vi "Redo.vi"(8 "error in (no error)":errorcluster, 11 "UndoObject in":refnum<class "UndoObject.lvclass">) -> (0 "error out":errorcluster, 2 "Ctrl Val.Get All":T1[](array[typedef]), 3 "UndoObject out":refnum<class "UndoObject.lvclass">, 4 "Redo Enable":bool, 6 "Undo Enable":bool)   [LabVIEW 2015, in "UndoLibrary.lvlib" / "UndoObject.lvclass"]
doc: "This VI stores the values to perform the redo action."
uses:
  UndoObject.lvclass
  Support VIs/DataClass/Controls/cluster_Control Value.ctl
  UndoObject.lvclass/UndoObject.ctl
  Support VIs/DataClass/DataObject.lvclass/DataObject.ctl
  QueueOperations/QueueOperations.lvlib
  Support VIs/DataClass/DataObject.lvclass
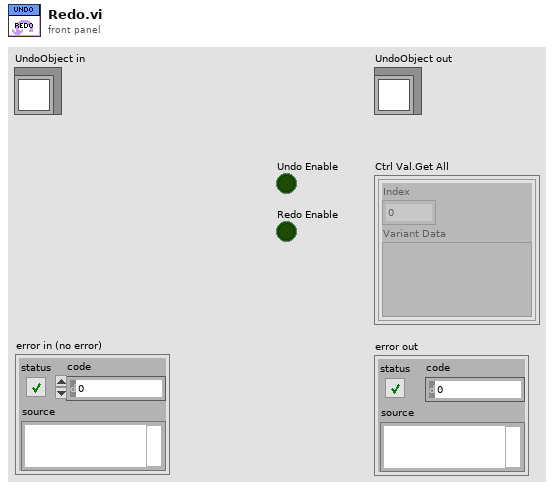
[diagram p1: front panel]
types:
  T1 = typedef "UndoLibrary.lvlib/DataObject.lvclass/cluster_Control Value.ctl" = cluster{"Index":i32, "Variant Data":variant}
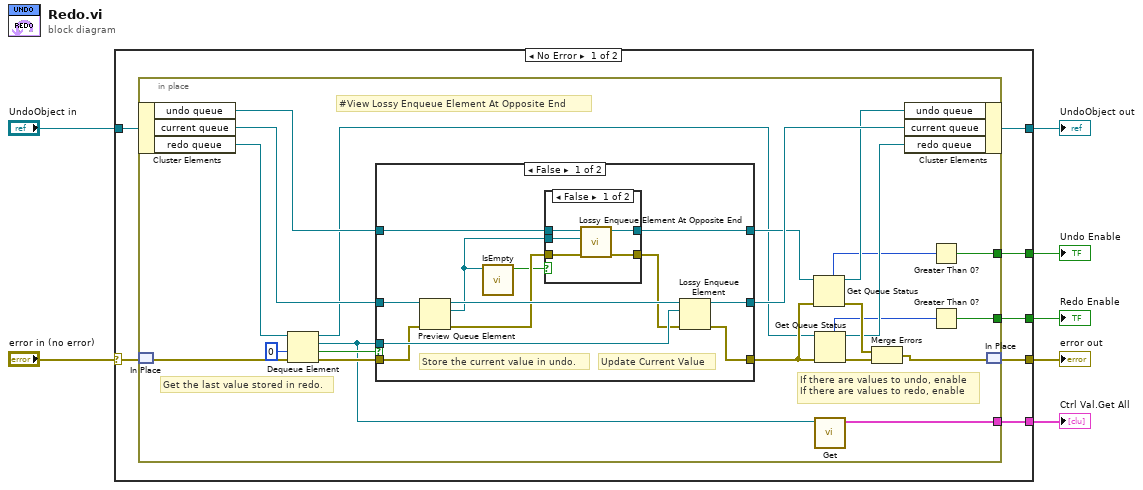
[diagram p0: block diagram]
diagram:
  n1 = case shown="No Error" "error in (no error)" {
    selector: "error in (no error)" -> [w13 w60]
    tunnel: [w12 w60] -> w7
    tunnel: "UndoObject in" -> [w11 w59]
    tunnel: [w14 _] -> w5
    tunnel: [w10 w59] -> w1
    tunnel: [w9 _] -> w4
    tunnel: [w8 _] -> w3
    frame No Error {
      n2 = in-place {
        in-place-border: [w15] -> w14
        in-place-border: [w19] -> w9
        in-place-border: [w17] -> w8
        # "Get the last value stored in redo."
        # "If there are values to undo, enable\nIf there are values to redo, enable"
        # "#View Lossy Enqueue Element At Opposite End"
        n3 = in-place-cluster #1(w11) -> ("undo queue"=w32:refnum<queue>, "current queue"=w31:refnum<queue>, "redo queue"=w30:refnum<queue>)
        n4 = in-place-match #2(w13) -> (w33:errorcluster)
        n5 = Dequeue Element(queue=w30, timeout in ms (-1)=0, error in (no error)=w33) -> (queue out=w22:refnum<queue>, element=w16:refnum<class "DataObject.lvclass">, timed out?=w35:bool, error out=w36:errorcluster)
        n6 = case shown="False" w35 {
          tunnel: w32 -> [w48 w58]
          tunnel: [w47 w58] -> w26
          tunnel: w36 -> [w41 w56]
          tunnel: w16 -> [w44 _]
          tunnel: w31 -> [w46 w57]
          tunnel: [w43 w57] -> w29
          tunnel: [w42 w56] -> w24
          frame False {
            # "Store the current value in undo."
            # "Update Current Value"
            n7 = Preview Queue Element(queue=w46, error in (no error)=w41) -> (queue out=w45:refnum<queue>, element=w37:refnum<class "DataObject.lvclass">, error out=w40:errorcluster)  [unwired: 1 in, 1 out]
            n8 = call "IsEmpty.vi"("DataObject in"=w37) -> ("empty?"=w38:bool)  [unwired: 9 in, 1 out]
            n9 = case shown="False" w38 {
              tunnel: w48 -> [w53 w54]
              tunnel: [w49 w54] -> w47
              tunnel: [w50 w55] -> w39
              tunnel: w40 -> [w51 w55]
              tunnel: w37 -> [w52 _]
              frame False {
                n10 = call "Lossy Enqueue Element At Opposite End.vi"("error in (no error)"=w51, "element"=w52, "queue in"=w53) -> ("error out"=w50:errorcluster, "queue out"=w49:refnum<queue>)  [unwired: 5 in, 2 out]
              }
              frame True {
              }
            }
            n11 = Lossy Enqueue Element(queue=w45, element=w44, error in (no error)=w39) -> (queue out=w43:refnum<queue>, error out=w42:errorcluster)  [unwired: 2 out]
          }
          frame True {
          }
        }
        n12 = Get Queue Status(queue=w26, error in (no error)=w24) -> (queue out=w25:refnum<queue>, error out=w27:errorcluster, # elements in queue=w20:i32)  [unwired: 1 in, 5 out]
        n13 = Get Queue Status(queue=w22, error in (no error)=w24) -> (queue out=w21:refnum<queue>, error out=w28:errorcluster, # elements in queue=w18:i32)  [unwired: 1 in, 5 out]
        n14 = call "Get.vi"("DataObject in"=w16) -> ("Conrol Value[]"=w15:T1[])  [unwired: 9 in, 1 out]
        n15 = Merge Errors(w27, w28) -> (w23:errorcluster)
        n16 = in-place-cluster #1("undo queue"=w25, "current queue"=w29, "redo queue"=w21) -> (w10:refnum<class "UndoObject.lvclass">)
        n17 = Greater Than 0?(x=w20) -> (x > 0?=w19:bool)
        n18 = Greater Than 0?(x=w18) -> (x > 0?=w17:bool)
        n19 = in-place-match #2(w23) -> (w12:errorcluster)
      }
    }
    frame Error {
    }
  }
  "error out" <- w7
  "Ctrl Val.Get All" <- w5
  "Undo Enable" <- w4
  "Redo Enable" <- w3
  "UndoObject out" <- w1
